vi "Get Compiled Counter And Protection Frames.vi"(0 "XNET Cluster":refnum<k21>, 5 "GUIDs":T9, 7 "Frames per type":T10[](array[typedef]) {"Frame Settings"."Transmit Trigger Ref" format="%.0x"; "Frame Settings"."Disable Transmission Ref" format="%.0x"; "Frame Refs" format="%.0x"}, 11 "error in (no error)":errorcluster) -> (4 "Frames":T2[](array[typedef]) {"Protection Configurations"."CRC Channels"."Data Type" items=["Signed", "Unsigned", "IEEE Float"]}, 6 "Signals Refs":T1[](array[typedef]) format="%.0x", 8 "Counters and Protection Refs":T1[](array[typedef]) format="%.0x", 10 "Override Refs":T1[](array[typedef]) format="%.0x", 15 "error out":errorcluster)   [LabVIEW 2024, in "Protection and Counter Support System Explorer.lvlib"]
uses:
  Protection and Counter Support System Explorer.lvlib
  Types/Export Frames List and Type.ctl
  Shared/Types/Exported Frame Type.ctl
  <vilib>/NI VeriStand/Custom Device API/Custom Device Item Ref.ctl
  Types/Exported Frame Settings.ctl
  Shared/Types/Exported Event Trigger Type.ctl
  Types/Export Frame GUIDs List.ctl
  Shared/Types/Exported Frame Settings.ctl
  Shared/Types/Exported Protection Settings.ctl
  Shared/Types/Protection Type.ctl
  Shared/Types/XNET Signal Configuration.ctl
  Shared/Types/Exported Counter Settings.ctl
  <vilib>/NI VeriStand/Custom Device Tools/Custom Device Utility Library/NI VeriStand - Search for All Items by GUID.vi
  Shared/Protection and Counter Support Shared.lvlib
  <vilib>/NI VeriStand/Custom Device API/Custom Device API.lvlib
  <resource>/objmgr/xnet.rc
  <vilib>/NI VeriStand/Custom Device Tools/Custom Device Utility Library/Custom Device Utility Library.lvlib
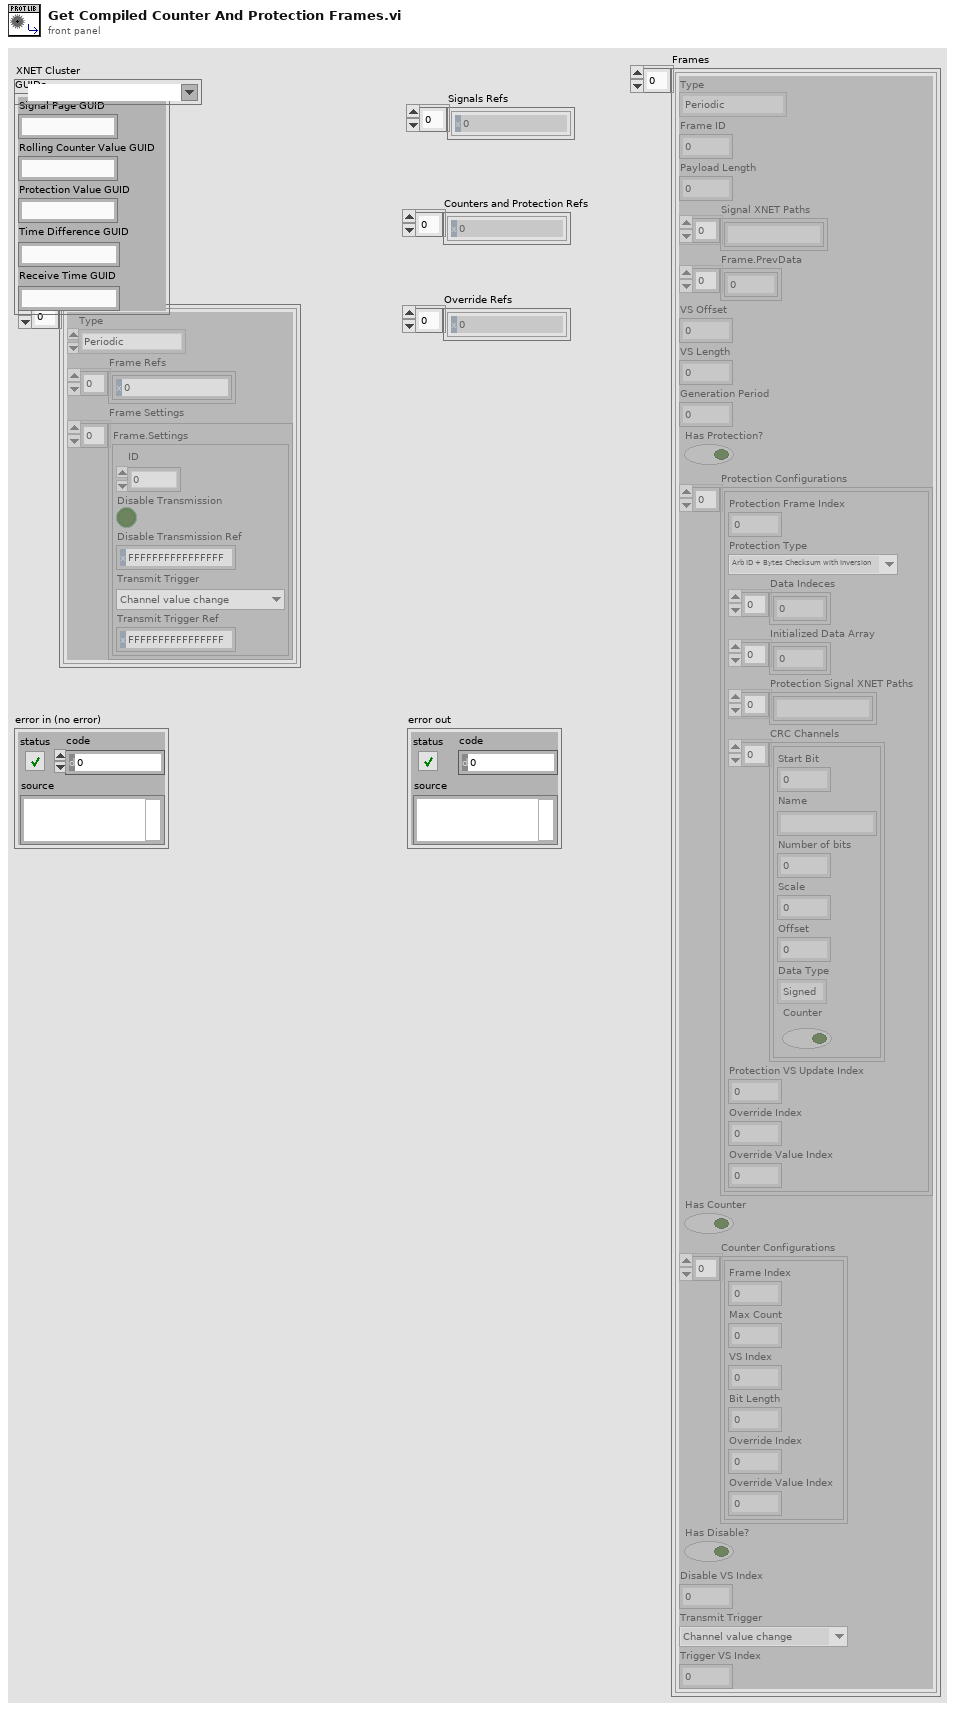
[diagram p1: front panel]
types:
  T1 = typedef "Custom Device API.lvlib/Custom Device Item Ref.ctl" = u64
  T2 = typedef "Protection and Counter Support Shared.lvlib/Exported Frame Settings.ctl" = cluster{"Type":T3, "Frame ID":u32, "Payload Length":u32, "Signal XNET Paths":string[], "Frame.PrevData":dbl[], "VS Offset":i32, "VS Length":i32, "Generation Period":u32, "Has Protection?":bool, "Protection Configurations":T4[], "Has Counter":bool, "Counter Configurations":T7[], "Has Disable?":bool, "Disable VS Index":i32, "Transmit Trigger":T8, "Trigger VS Index":i32}
  T3 = typedef "Protection and Counter Support Shared.lvlib/Exported Frame Type.ctl" = enum16{"Periodic", "Event", "Periodic/Event"}
  T4 = typedef "Protection and Counter Support Shared.lvlib/Exported Protection Settings.ctl" = cluster{"Protection Frame Index":i32, "Protection Type":T5, "Data Indeces":i32[], "Initialized Data Array":dbl[], "Protection Signal XNET Paths":string[], "CRC Channels":T6[], "Protection VS Update Index":i32, "Override Index":i32, "Override Value Index":i32}
  T5 = typedef "Protection and Counter Support Shared.lvlib/Protection Type.ctl" = enum16{"Arb ID + Bytes Checksum with Inversion", "Arb ID + Bytes CRC with Inversion", "Reversed Raw Signal Checksum with Inversion", "Concatenated Two's Compliment"}
  T6 = typedef "Protection and Counter Support Shared.lvlib/XNET Signal Configuration.ctl" = cluster{"Start Bit":i32, "Name":string, "Number of bits":i32, "Scale":dbl, "Offset":dbl, "Data Type":u32, "Counter":bool}
  T7 = typedef "Protection and Counter Support Shared.lvlib/Exported Counter Settings.ctl" = cluster{"Frame Index":i32, "Max Count":dbl, "VS Index":i32, "Bit Length":i64, "Override Index":i32, "Override Value Index":i32}
  T8 = typedef "Protection and Counter Support Shared.lvlib/Exported Event Trigger Type.ctl" = enum16{"Channel value change", "Trigger channel (not zero)", "Channel value change or trigger channel (not zero)", "Trigger channel (any value change)", "Channel value change or trigger channel (any value change)"}
  T9 = typedef "Protection and Counter Support System Explorer.lvlib/Export Frame GUIDs List.ctl" = cluster{"Signal Page GUID":string, "Rolling Counter Value GUID":string, "Protection Value GUID":string, "Time Difference GUID":string, "Receive Time GUID":string}
  T10 = typedef "Protection and Counter Support System Explorer.lvlib/Export Frames List and Type.ctl" = cluster{"Type":T3, "Frame Refs":T1[], "Frame Settings":T11[]}
  T11 = typedef "Protection and Counter Support System Explorer.lvlib/Exported Frame Settings.ctl" = cluster{"ID":u32, "Disable Transmission":bool, "Disable Transmission Ref":T1, "Transmit Trigger":T8, "Transmit Trigger Ref":T1}
  T12 = typedef "Custom Device API.lvlib/Custom Device Item Info.ctl" = cluster{"Name":string, "Is Channel":bool, "GUID":string, "Is Waveform":bool}
  T13 = typedef "Protection and Counter Support System Explorer.lvlib/Protection Signal Settings.ctl" = cluster{"Input Channels":T14[], "Protection Type":T5}
  T14 = typedef "Protection and Counter Support System Explorer.lvlib/Protection Signal Linked Channel.ctl" = cluster{"Node Ref":T1}
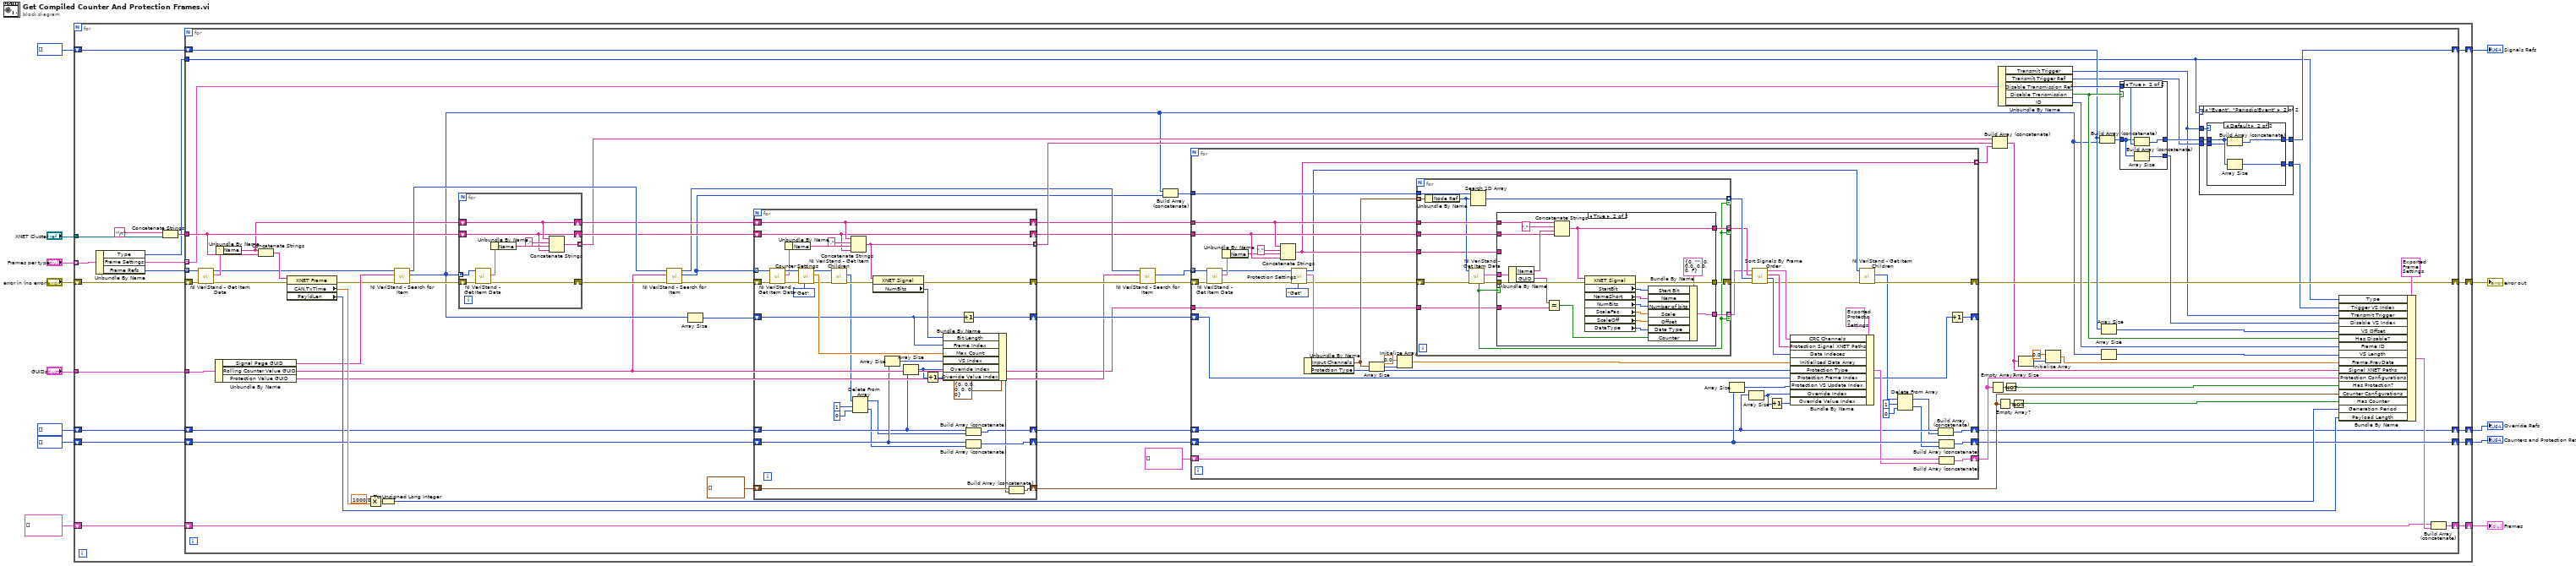
[diagram p0: block diagram]
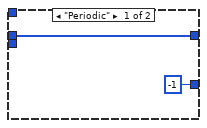
[diagram p2: hidden frame]
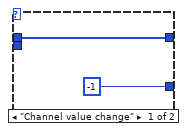
[diagram p3: hidden frame]
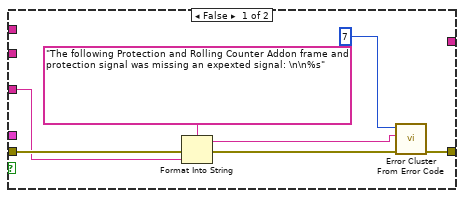
[diagram p4: hidden frame]
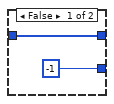
[diagram p5: hidden frame]
diagram:
  n1 = for {
    tunnel: "XNET Cluster" -> [w31]
    shift-right: [w26] -> w1
    shift-left: "error in (no error)" -> [w20]
    shift-right: [w25] -> w7
    shift-left: T2[] [] -> [w24]
    shift-right: [w28] -> w5
    shift-left: T1[] [] -> [w23]
    shift-right: [w27] -> w6
    shift-left: T1[] [] -> [w22]
    tunnel: "GUIDs" -> [w21]
    tunnel: "Frames per type" -> [w19] mode=indexing
    shift-right: [w14] -> w2
    shift-left: T1[] [] -> [w15]
    n2 = Unbundle By Name(w19) -> ("Type"=w18:T3, "Frame Settings"=w16:T11[], "Frame Refs"=w17:T1[])
    n3 = Concatenate Strings("\n", w31) -> (w29:string)
    n4 = for {
      tunnel: w17 -> [w90] mode=indexing
      shift-right: [w59] -> w26
      shift-left: w20 -> [w91]
      shift-right: [w102] -> w28
      shift-left: w23 -> [w100]
      tunnel: w29 -> [w75]
      shift-right: [w53] -> w27
      shift-left: w22 -> [w81]
      shift-right: [w44] -> w25
      shift-left: w24 -> [w43]
      tunnel: w18 -> [w42]
      tunnel: w21 -> [w41]
      tunnel: w16 -> [w38] mode=indexing
      shift-right: [w32] -> w14
      shift-left: w15 -> [w34]
      n5 = call <vilib>:"NI VeriStand - Get Item Data.vi"("error in (no error)"=w91, "Item Ref in"=w90) -> ("error out"=w87:errorcluster, "Item Info"=w89:T12, "Item Ref out"=w36:T1)  [unwired: 6 in, 1 out]
      n6 = Unbundle By Name(w41) -> ("Signal Page GUID"=w40:string, "Rolling Counter Value GUID"=w35:string, "Protection Value GUID"=w39:string)
      n7 = Unbundle By Name(w89) -> ("Name"=w74:string)
      n8 = Concatenate Strings(w74, w75) -> (w88:string)
      n9 = property class="XNET Frame"(reference=w88, error in=w87) -> (error out=w37:errorcluster, "CAN.TxTime"=w85:dbl, "PayldLen"=w49:u32)  [unwired: 1 out]
      n10 = Multiply(x=1000.0 ("y"), y=w85) -> (x*y=w86:dbl)
      n11 = To Unsigned Long Integer(number=w86) -> (unsigned 32bit integer=w83:u32)
      n12 = call-poly <vilib>:"NI VeriStand - Search for Item.vi"("error in"=w37, "Item GUID"=w40, "Section Ref in"=w36) -> ("error out"=w77:errorcluster, "Item Refs"=w51:T1[], "Section Ref out"=w80:T1)  [unwired: 5 in, 1 out]
      n13 = for {
        tunnel: w51 -> [w218] mode=indexing
        shift-right: [w212] -> w76
        shift-left: w77 -> [w217]
        tunnel: [w214] -> w71 mode=indexing
        shift-right: [w211] -> w73
        shift-left: w74 -> [w211]
        shift-right: [w210] -> w72
        shift-left: w75 -> [w210]
        n14 = call <vilib>:"NI VeriStand - Get Item Data.vi"("error in (no error)"=w217, "Item Ref in"=w218) -> ("error out"=w212:errorcluster, "Item Info"=w213:T12)  [unwired: 6 in, 2 out]
        n15 = Unbundle By Name(w213) -> ("Name"=w215:string)
        n16 = Concatenate Strings(w211, "." ("string"), w215, w210) -> (w214:string)
      }
      n17 = call-poly <vilib>:"NI VeriStand - Search for Item.vi"("error in"=w76, "Item GUID"=w35, "Section Ref in"=w80) -> ("error out"=w79:errorcluster, "Item Refs"=w50:T1[], "Section Ref out"=w68:T1)  [unwired: 5 in, 1 out]
      n18 = Array Size(array=w51) -> (size(s)=w78:i32)
      n19 = for {
        tunnel: w50 -> [w253] mode=indexing
        shift-right: [w234] -> w69
        shift-left: w79 -> [w252]
        shift-right: [w249] -> w92
        shift-left: T7[] [] -> [w248]
        tunnel: [w233] -> w70 mode=indexing
        shift-right: [w243] -> w54
        shift-left: w81 -> [w244]
        shift-right: [w238] -> w64
        shift-left: w78 -> [w231]
        shift-right: [w237] -> w62
        shift-left: w73 -> [w237]
        shift-right: [w236] -> w63
        shift-left: w72 -> [w236]
        shift-right: [w225] -> w33
        shift-left: w34 -> [w230]
        n20 = call <vilib>:"NI VeriStand - Get Item Data.vi"("error in (no error)"=w252, "Item Ref in"=w253) -> ("error out"=w250:errorcluster, "Item Info"=w245:T12, "Item Ref out"=w251:T1)  [unwired: 6 in, 1 out]
        n21 = Unbundle By Name(w245) -> ("Name"=w246:string)
        n22 = call "Counter Settings.vi"("Action"=enum8{"Get", "Set"}."Get", "error in"=w250, "Parent Ref"=w251) -> ("error out"=w227:errorcluster, "Max Count"=w242:dbl, "Parent Ref Out"=w222:T1)  [unwired: 6 in]
        n23 = call <vilib>:"NI VeriStand - Get Item Children.vi"("error in (no error)"=w227, "Item Ref in"=w222) -> ("error out"=w226:errorcluster, "Child Refs"=w220:T1[])  [unwired: 6 in, 2 out]
        n24 = Concatenate Strings(w237, "." ("string"), w246, w236) -> (w233:string)
        n25 = Delete From Array(array=w220, length=1, index=0) -> (deleted portion=w221:T1[], array with subset deleted=w219:T1[])
        n26 = property class="XNET Signal"(reference=w233, error in=w226) -> (error out=w234:errorcluster, "NumBits"=w232:u32)  [unwired: 1 out]
        n27 = Array Size(array=w244) -> (size(s)=w239:i32)
        n28 = Array Size(array=w230) -> (size(s)=w229:i32)
        n29 = Increment(x=w229) -> (x+1=w228:i32)
        n30 = Bundle By Name(cluster=T7 {"Frame Index"=0, "Max Count"=0.0, "VS Index"=0, "Bit Length"=0, "Override Index"=0, "Override Value Index"=0} ("Cluster"), "Bit Length"=w232, "Frame Index"=w231, "Max Count"=w242, "VS Index"=w239, "Override Index"=w229, "Override Value Index"=w228) -> (w241:T7)
        n31 = Increment(x=w231) -> (x+1=w238:i32)
        n32 = Build Array (concatenate)(w230, w219) -> (w225:T1[])
        n33 = Build Array (concatenate)(w244, w221) -> (w243:T1[])
        n34 = Build Array (concatenate)(w248, w241) -> (w249:T7[])
      }
      n35 = call-poly <vilib>:"NI VeriStand - Search for Item.vi"("error in"=w69, "Item GUID"=w39, "Section Ref in"=w68) -> ("error out"=w67:errorcluster, "Item Refs"=w66:T1[])  [unwired: 5 in, 2 out]
      n36 = Build Array (concatenate)(w51, w50) -> (w52:T1[])
      n37 = for {
        tunnel: w66 -> [w168] mode=indexing
        shift-right: [w127] -> w59
        shift-left: w67 -> [w167]
        shift-right: [w164] -> w60
        shift-left: T4[] [] -> [w166]
        tunnel: w52 -> [w165]
        tunnel: w62 -> [w162]
        tunnel: [w144] -> w61 mode=indexing
        shift-right: [w158] -> w53
        shift-left: w54 -> [w159]
        shift-right: [w146] -> _
        shift-left: w64 -> [w147]
        tunnel: w63 -> [w161]
        tunnel: w35 -> [w142]
        shift-right: [w132] -> w32
        shift-left: w33 -> [w131]
        n38 = call <vilib>:"NI VeriStand - Get Item Data.vi"("error in (no error)"=w167, "Item Ref in"=w168) -> ("error out"=w130:errorcluster, "Item Info"=w160:T12, "Item Ref out"=w129:T1)  [unwired: 6 in, 1 out]
        n39 = Unbundle By Name(w160) -> ("Name"=w145:string)
        n40 = Concatenate Strings(w162, "." ("string"), w145, w161) -> (w144:string)
        n41 = call "Protection Settings.vi"("Action"=enum8{"Get", "Set"}."Get", "error in"=w130, "Parent Ref"=w129) -> ("error out"=w150:errorcluster, "Selected Channels"=w157:T13, "Parent Ref Out"=w126:T1)  [unwired: 6 in]
        n42 = Unbundle By Name(w157) -> ("Input Channels"=w155:T14[], "Protection Type"=w156:T5)
        n43 = Array Size(array=w155) -> (size(s)=w154:i32)
        n44 = Initialize Array(0.0 ("element"), w154) -> (w152:dbl[])
        n45 = for {
          tunnel: w165 -> [w173]
          tunnel: w155 -> [w183] mode=indexing
          tunnel: [w182] -> w141 mode=indexing if=w171
          shift-right: [w176] -> w139
          shift-left: w150 -> [w181]
          tunnel: w162 -> [w179]
          tunnel: w161 -> [w178]
          tunnel: [w174] -> w138 mode=indexing if=w171
          tunnel: [w175] -> w137 mode=indexing if=w171
          tunnel: w144 -> [w170]
          tunnel: w142 -> [w169]
          n46 = Unbundle By Name(w183) -> ("Node Ref"=w172:T1)
          n47 = call <vilib>:"NI VeriStand - Get Item Data.vi"("error in (no error)"=w181, "Item Ref in"=w172) -> ("error out"=w177:errorcluster, "Item Info"=w180:T12, "Found"=w171:bool)  [unwired: 6 in, 1 out]
          n48 = Search 1D Array(1D array=w173, element=w172) -> (index of element=w182:i32)  [unwired: 1 in]
          n49 = case shown="True" w171 {
            tunnel: w180 -> [_ w209]
            tunnel: w179 -> [_ w206]
            tunnel: w178 -> [_ w205]
            tunnel: w177 -> [w188 w204]
            tunnel: [w190 w203] -> w176
            tunnel: [_ w195] -> w175
            tunnel: [_ w194] -> w174
            tunnel: w170 -> [w185 _]
            tunnel: w169 -> [_ w193]
            frame False {
              n50 = Format Into String(format string="The following Protection and Rolling Counter Addon frame and protection signal was missing an expexted signal: \n\n%s" ("error message (\"\")"), error in=w188, w185) -> (resulting string=w184:string, error out=w187:errorcluster)  [unwired: 1 in]
              n51 = call <vilib>:"Error Cluster From Error Code.vi"("error in (no error)"=w187, "error message (\"\")"=w184, "error code (0)"=7) -> ("error out"=w190:errorcluster)  [unwired: 6 in]
            }
            frame True {
              n52 = Unbundle By Name(w209) -> ("Name"=w207:string, "GUID"=w191:string)
              n53 = Equal?(x=w191, y=w193) -> (x = y?=w192:bool)
              n54 = Concatenate Strings(w206, "." ("string"), w207, w205) -> (w194:string)
              n55 = property class="XNET Signal"(reference=w194, error in=w204) -> (error out=w203:errorcluster, "StartBit"=w196:u32, "NameShort"=w197:string, "NumBits"=w198:u32, "ScaleFac"=w199:dbl, "ScaleOff"=w200:dbl, "DataType"=w201:u32)  [unwired: 1 out]
              n56 = Bundle By Name(cluster=T6 {"Start Bit"=0, "Name"="", "Number of bits"=0, "Scale"=0.0, "Offset"=0.0, "Data Type"=0, "Counter"=FALSE} ("MonitoredChannelSettings"), "Start Bit"=w196, "Name"=w197, "Number of bits"=w198, "Scale"=w199, "Offset"=w200, "Data Type"=w201, "Counter"=w192) -> (w195:T6)
            }
          }
        }
        n57 = Array Size(array=w159) -> (size(s)=w148:i32)
        n58 = Array Size(array=w131) -> (size(s)=w134:i32)
        n59 = call "Sort Signals By Frame Order.vi"("error in (no error)"=w139, "Node Refs"=w141, "XNET Paths"=w138, "Signals"=w137) -> ("error out"=w128:errorcluster, "Ordered Node Refs"=w140:i32[], "Ordered XNET Paths"=w135:string[], "Ordered Signals"=w136:T6[])  [unwired: 4 in]
        n60 = Increment(x=w134) -> (x+1=w133:i32)
        n61 = Bundle By Name(cluster=T4 {"Protection Frame Index"=0, "Protection Type"=enum."Arb ID + Bytes Checksum with Inversion", "Data Indeces"=[], "Initialized Data Array"=[], "Protection Signal XNET Paths"=[], "CRC Channels"=[], "Protection VS Update Index"=0, "Override Index"=0, "Override Value Index"=0} ("Cluster"), "CRC Channels"=w136, "Protection Signal XNET Paths"=w135, "Data Indeces"=w140, "Initialized Data Array"=w152, "Protection Type"=w156, "Protection Frame Index"=w147, "Protection VS Update Index"=w148, "Override Index"=w134, "Override Value Index"=w133) -> (w151:T4)
        n62 = call <vilib>:"NI VeriStand - Get Item Children.vi"("error in (no error)"=w128, "Item Ref in"=w126) -> ("error out"=w127:errorcluster, "Child Refs"=w122:T1[])  [unwired: 6 in, 2 out]
        n63 = Delete From Array(array=w122, length=1, index=0) -> (deleted portion=w123:T1[], array with subset deleted=w121:T1[])
        n64 = Build Array (concatenate)(w131, w121) -> (w132:T1[])
        n65 = Build Array (concatenate)(w159, w123) -> (w158:T1[])
        n66 = Build Array (concatenate)(w166, w151) -> (w164:T4[])
        n67 = Increment(x=w147) -> (x+1=w146:i32)
      }
      n68 = Empty Array?(array=w60) -> (empty?=w94:bool)
      n69 = Build Array (concatenate)(w71, w70, w61) -> (w58:string[])
      n70 = Empty Array?(array=w92) -> (empty?=w96:bool)
      n71 = Unbundle By Name(w38) -> ("Transmit Trigger"=w47:T8, "Transmit Trigger Ref"=w48:T1, "Disable Transmission Ref"=w104:T1, "Disable Transmission"=w105:bool, "ID"=w106:u32)
      n72 = Not(x=w94) -> (.not. x?=w93:bool)
      n73 = Not(x=w96) -> (.not. x?=w95:bool)
      n74 = Array Size(array=w58) -> (size(s)=w56:i32)
      n75 = Initialize Array(0.0 ("element"), w56) -> (w55:dbl[])
      n76 = Build Array (concatenate)(w100, w51) -> (w101:T1[])
      n77 = Array Size(array=w100) -> (size(s)=w99:i32)
      n78 = Array Size(array=w51) -> (size(s)=w82:i32)
      n79 = case shown="True" w105 {
        tunnel: w101 -> [w255 w257]
        tunnel: [w255 w259] -> w103
        tunnel: w104 -> [_ w258]
        tunnel: [-1 w256] -> w98
        frame False {
        }
        frame True {
          n80 = Build Array (concatenate)(w257, w258) -> (w259:T1[])
          n81 = Array Size(array=w257) -> (size(s)=w256:i32)
        }
      }
      n82 = case shown="\"Event\", \"Periodic/Event\"" w42 {
        tunnel: w103 -> [w109 w114]
        tunnel: [w109 w113] -> w102
        tunnel: w48 -> [_ w112]
        tunnel: w47 -> [_ w111]
        tunnel: [-1 w110] -> w46
        frame "Periodic" {
        }
        frame "Event", "Periodic/Event" {
          n83 = case shown="Default" w111 {
            tunnel: w114 -> [w116 w119]
            tunnel: [w116 w120] -> w113
            tunnel: [-1 w118] -> w110
            tunnel: w112 -> [_ w117]
            frame "Channel value change" {
            }
            frame Default {
              n84 = Array Size(array=w119) -> (size(s)=w118:i32)
              n85 = Build Array (concatenate)(w119, w117) -> (w120:T1[])
            }
          }
        }
      }
      n86 = Bundle By Name(cluster=T2 {"Type"=enum."Periodic", "Frame ID"=0, "Payload Length"=0, "Signal XNET Paths"=[], "Frame.PrevData"=[], "VS Offset"=0, "VS Length"=0, "Generation Period"=0, "Has Protection?"=FALSE, "Protection Configurations"=[], "Has Counter"=FALSE, "Counter Configurations"=[], "Has Disable?"=FALSE, "Disable VS Index"=0, "Transmit Trigger"=enum."Channel value change", "Trigger VS Index"=0} ("Frame Settings"), "Type"=w42, "Trigger VS Index"=w46, "Transmit Trigger"=w47, "Disable VS Index"=w98, "VS Offset"=w99, "Has Disable?"=w105, "Frame ID"=w106, "VS Length"=w82, "Frame.PrevData"=w55, "Signal XNET Paths"=w58, "Protection Configurations"=w60, "Has Protection?"=w93, "Counter Configurations"=w92, "Has Counter"=w95, "Generation Period"=w83, "Payload Length"=w49) -> (w45:T2)
      n87 = Build Array (concatenate)(w43, w45) -> (w44:T2[])
    }
  }
  "Frames" <- w7
  "error out" <- w1
  "Counters and Protection Refs" <- w6
  "Signals Refs" <- w5
  "Override Refs" <- w2
